vi "add filename to protocol notes.vi"(11 "rec start/end (T is start)":bool) -> (3 "protocol.notes out":string)   [LabVIEW 2012]
doc: "SciScan 1.2 160622"
uses:
  GFG/GFGstringGet.vi
  GFG/GFGpathGet.vi
  GFG/GFGfpRefGet.vi
  GFG/GFG library.lvlib
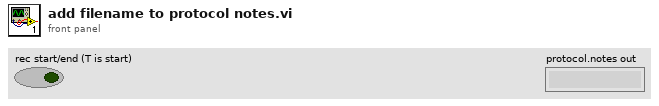
[diagram p1: front panel]
types:
  T1 = cluster{"WaveformChartRef":refnum<vi>, "DigitalRef":refnum<vi>, "ArrayRef":refnum<vi>, "TabControlRef":refnum<vi>, "EnumRef":refnum<vi>, "RingRef":refnum<vi>, "BooleanRef":refnum<vi>, "KnobRef":refnum<vi>, "SlideRef":refnum<vi>, "PathRef":refnum<vi>, "StringRef":refnum<vi>, "ComboBox":refnum<vi>, "WaveformGraphRef":refnum<vi>}
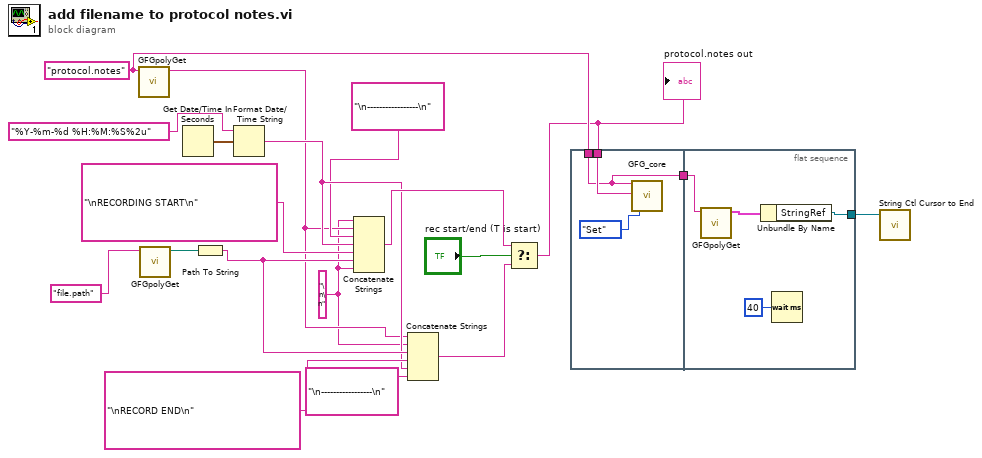
[diagram p0: block diagram]
diagram:
  w1 = "\n\n" ("string")
  w16 = "protocol.notes" ("Variable Name in")
  n1 = call-poly "GFGpolyGet.vi"("Variable Name in"=w16) -> ("String"=w2:string)  [unwired: 9 in, 1 out]
  n2 = call-poly "GFGpolyGet.vi"("Variable Name in"="file.path" ("Tag in")) -> ("Path"=w17:path)  [unwired: 8 in, 2 out]
  n3 = Get Date/Time In Seconds() -> (seconds since 1Jan1904=w6:timestamp)
  n4 = Path To String(path=w17) -> (string=w15:string)
  n5 = Format Date/Time String(time format string (%c)="%Y-%m-%d %H:%M:%S%2u", seconds (now)=w6) -> (date/time string=w4:string)  [unwired: 1 in]
  n6 = Concatenate Strings(w1, w2, "\n-----------------\n" ("string"), w4, "\nRECORDING START\n" ("string"), w15, w1) -> (w13:string)
  n7 = Concatenate Strings(w2, w1, w15, "\nRECORD END\n" ("string"), w4, "\n-----------------\n" ("string")) -> (w11:string)
  n8 = Select(t=w13, s="rec start/end (T is start)", f=w11) -> (s? t:f=w12:string)
  "protocol.notes out" <- w12
  n9 = flat-sequence {
    tunnel: w16 -> [w20]
    tunnel: w12 -> [w21]
    tunnel: [w20] -> w9
    tunnel: w9 -> [w26]
    tunnel: [w24] -> w8
    frame #0 {
      n10 = call "GFG_core.vi"("Variable Name in"=w20, "Variant in"=w21, "Action"=enum16{"Init", "Set", "Get"}."Set") -> ()  [unwired: 10 in, 7 out]
    }
    frame #1 {
      n11 = call-poly "GFGpolyGet.vi"("Variable Name in"=w26) -> ("output cluster"=w25:T1)  [unwired: 9 in, 1 out]
      n12 = Unbundle By Name(w25) -> ("StringRef"=w24:refnum<vi>)
      n13 = Wait (ms)(milliseconds to wait=u32 40) -> ()  [unwired: 1 out]
    }
  }
  n14 = call "String Ctl Cursor to End.vi"("String Reference in"=w8) -> ()  [unwired: 10 in, 1 out]
